vi "headless.vi"() -> ()   [LabVIEW 2026]
panel:
  out "time string":string
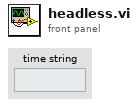
[diagram p1: front panel]
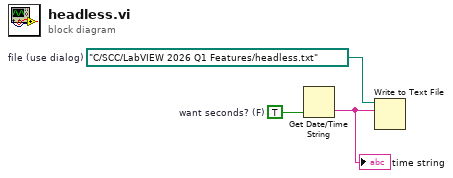
[diagram p0: block diagram]
diagram:
  w2 = path "C:/SCC/LabVIEW 2026 Q1 Features/headless.txt"  # file (use dialog)
  w3 = TRUE  # want seconds? (F)
  n1 = Get Date/Time String(want seconds? (F)=w3) -> (time string=w1:string)  [unwired: 2 in, 1 out]
  "time string" <- w1
  n2 = Write to Text File(file (use dialog)=w2, text=w1) -> ()  [unwired: 2 in, 3 out]
